vi "UNIX to Timenumber.vi"(1 "Seconds":i32) -> (0 "Timestamp String":string)   [LabVIEW 2009]
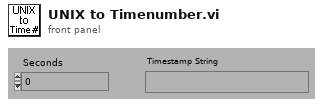
[diagram p1: front panel]
types:
  T1 = cluster{"second":i32, "minute":i32, "hour":i32, "day of month":i32, "month":i32, "year":i32, "day of week":i32, "day of year":i32, "is DST":i32}
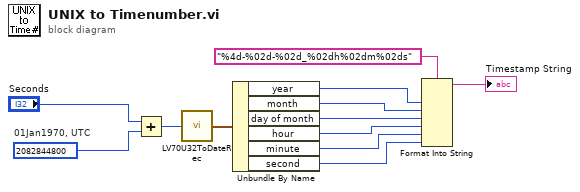
[diagram p0: block diagram]
diagram:
  w3 = 2082844800  # 01Jan1970, UTC
  n1 = Add(x="Seconds", y=w3) -> (x+y=w4:i32)
  n2 = call <vilib>:"LV70U32ToDateRec.vi"("Time"=w4) -> ("date time rec"=w12:T1)
  n3 = Unbundle By Name(w12) -> ("year"=w10:i32, "month"=w1:i32, "day of month"=w9:i32, "hour"=w8:i32, "minute"=w7:i32, "second"=w6:i32)
  n4 = Format Into String(format string="%4d-%02d-%02d_%02dh%02dm%02ds", w10, w1, w9, w8, w7, w6) -> (resulting string=→"Timestamp String":string)  [unwired: 2 in, 1 out]
